vi "H(f).vi"(1 "f":dbl format="%0.4e", 2 "N":i32, 3 "An":dbl[](array[numeric]) format="%0.2f") -> (0 "y":dbl format="%0.2f")   [LabVIEW 2010, in "NI_AALPro.lvlib"]
doc: "Computes the magnitude of the window's frequency response given the set of window coefficients and the size of the window in samples."
uses:
  NI_AALPro.lvlib
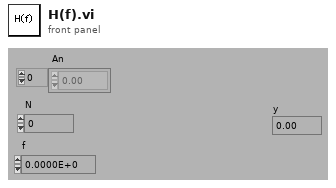
[diagram p1: front panel]
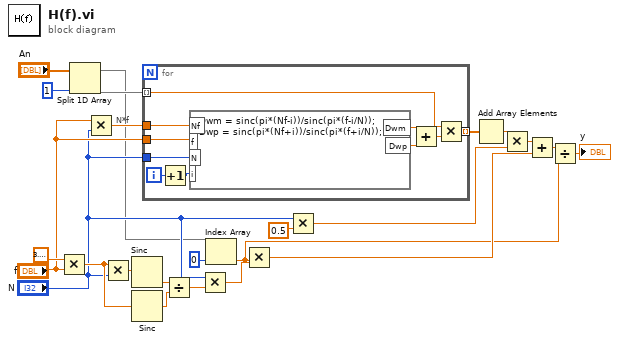
[diagram p0: block diagram]
diagram:
  # "N*f"
  n1 = Multiply(x=3.141592653589793, y="f") -> (x*y=w22:dbl)
  n2 = Split 1D Array(array="An", index=1) -> (first subarray=w1:dbl[], second subarray=w2:dbl[])
  n3 = Multiply(x="f", y="N") -> (x*y=w18:dbl)
  n4 = Multiply(x=w22, y="N") -> (x*y=w23:dbl)
  n5 = Sinc(1:w23) -> (0:w21:dbl)
  n6 = Sinc(1:w22) -> (0:w20:dbl)
  n7 = for {
    tunnel: "f" -> [w32]
    tunnel: w18 -> [w33]
    tunnel: [w28] -> w17 mode=indexing
    tunnel: "N" -> [w26]
    tunnel: w2 -> [w25] mode=indexing
    i -> [w34]
    n8 = Increment(x=w34) -> (x+1=w27:i32)
    n9 = formula code="Dwm = sinc(pi*(Nf-i))/sinc(pi*(f-i/N));\nDwp = sinc(pi*(Nf+i))/sinc(pi*(f+i/N));"("Nf"=w33, "f"=w32, "i"=w27, "N"=w26) -> ("Dwm"=w31:dbl, "Dwp"=w30:dbl)
    n10 = Add(x=w31, y=w30) -> (x+y=w29:dbl)
    n11 = Multiply(x=w25, y=w29) -> (x*y=w28:dbl)
  }
  n12 = Divide(x=w21, y=w20) -> (x/y=w11:dbl)
  n13 = Multiply(x="N", y=w11) -> (x*y=w12:dbl)
  n14 = Index Array(array=w1, index=0) -> (element=w5:dbl)
  n15 = Multiply(x=w5, y=w12) -> (x*y=w9:dbl)
  n16 = Multiply(x="N", y=0.5) -> (x*y=w15:dbl)
  n17 = Add Array Elements(numeric array=w17) -> (sum=w16:dbl)
  n18 = Multiply(x=w16, y=w15) -> (x*y=w10:dbl)
  n19 = Add(x=w10, y=w9) -> (x+y=w8:dbl)
  n20 = Divide(x=w8, y=w5) -> (x/y=→"y":dbl)
